vi "0 - Controle Xbox.vi"() -> (2 "R Thumb":i32(slide) scale=-32768.0..32768.0)   [LabVIEW 2020]
uses:
  <vilib>/robotics/Controls/Compass Indicator/Compass Indicator.xctl
  d73543a5-2c4f-4594-8cde-04c26e843dca.vi
  073897dc-bfc7-4ae1-a47e-8832abdac106.vi
  1fd616fa-7c11-4f18-9353-dc0f775eeb70.vi
  12afcf76-136b-4d38-a805-5952addfd333.vi
  20e97823-944d-452c-9f5c-32b38a6acdda.vi
  48340986-43e5-49c4-9512-bc3a2c788b05.vi
  cd7113f7-14d5-4977-ab3b-8115f77a9605.vi
  7e22e7d3-76e1-429a-a868-e97800e19938.vi
  749baf19-c05a-4ab2-9a75-a53bd8d5225c.vi
  9b3ce3fb-1892-4e24-a592-ce18c55ace7c.vi
  <vilib>/picture/3D Picture Control/Object/Create Object (drawable).vi
  <vilib>/Utility/inputDevices.llb/joystickAcquire.vi
  <vilib>/Utility/inputDevices.llb/closeJoystick.vi
  <vilib>/picture/3D Picture Control/NI_3D Picture Control.lvlib
panel:
  in  "Relative?":bool
  in  "Color":T1={"Red"=1.0, "Green"=0.0, "Blue"=0.0, "Alpha"=1.0}
  out "3D Picture":refnum<vi>(3d-picture)
  out "Garra Acionada":bool
  out "Slide 2":u8(slide) caption="Avanço da Garra" scale=0.0..100.0
  out "Slide":u8(slide) caption="Rotação"
  out "Altura 1":bool
  out "Altura 2":bool
  out "Altura 3":bool
  out "número 4":i32 caption="Y (apertar)"
  out "número 3":i32 caption="X (segurar)"
  out "número 2":i32 caption="B (soltar)"
  out "número":i32 caption="A (1-2-3)"
  out "Analógico Direito":dbl(xcontrol)
  out "Analógico Esquerdo":dbl(xcontrol)
  out "Start":bool
  out "Stop/Back":bool
  out "Right trigger":bool
  out "Left Trigger":bool
  out "Cluster":T2
  out "LThumb":i32(slide) scale=-32768.0..32768.0
  out "Left Thumb button":bool
  out "Right Thumb button":bool
  out "LB":bool
  out "RB":bool
  out "Y":bool
  out "X":bool
  out "B":bool
  out "A":bool caption="Boolean"
  out "joystick info":T3(array[cluster])
  out "direction info":T4
  out "button info":T5
  out "axis info":T6
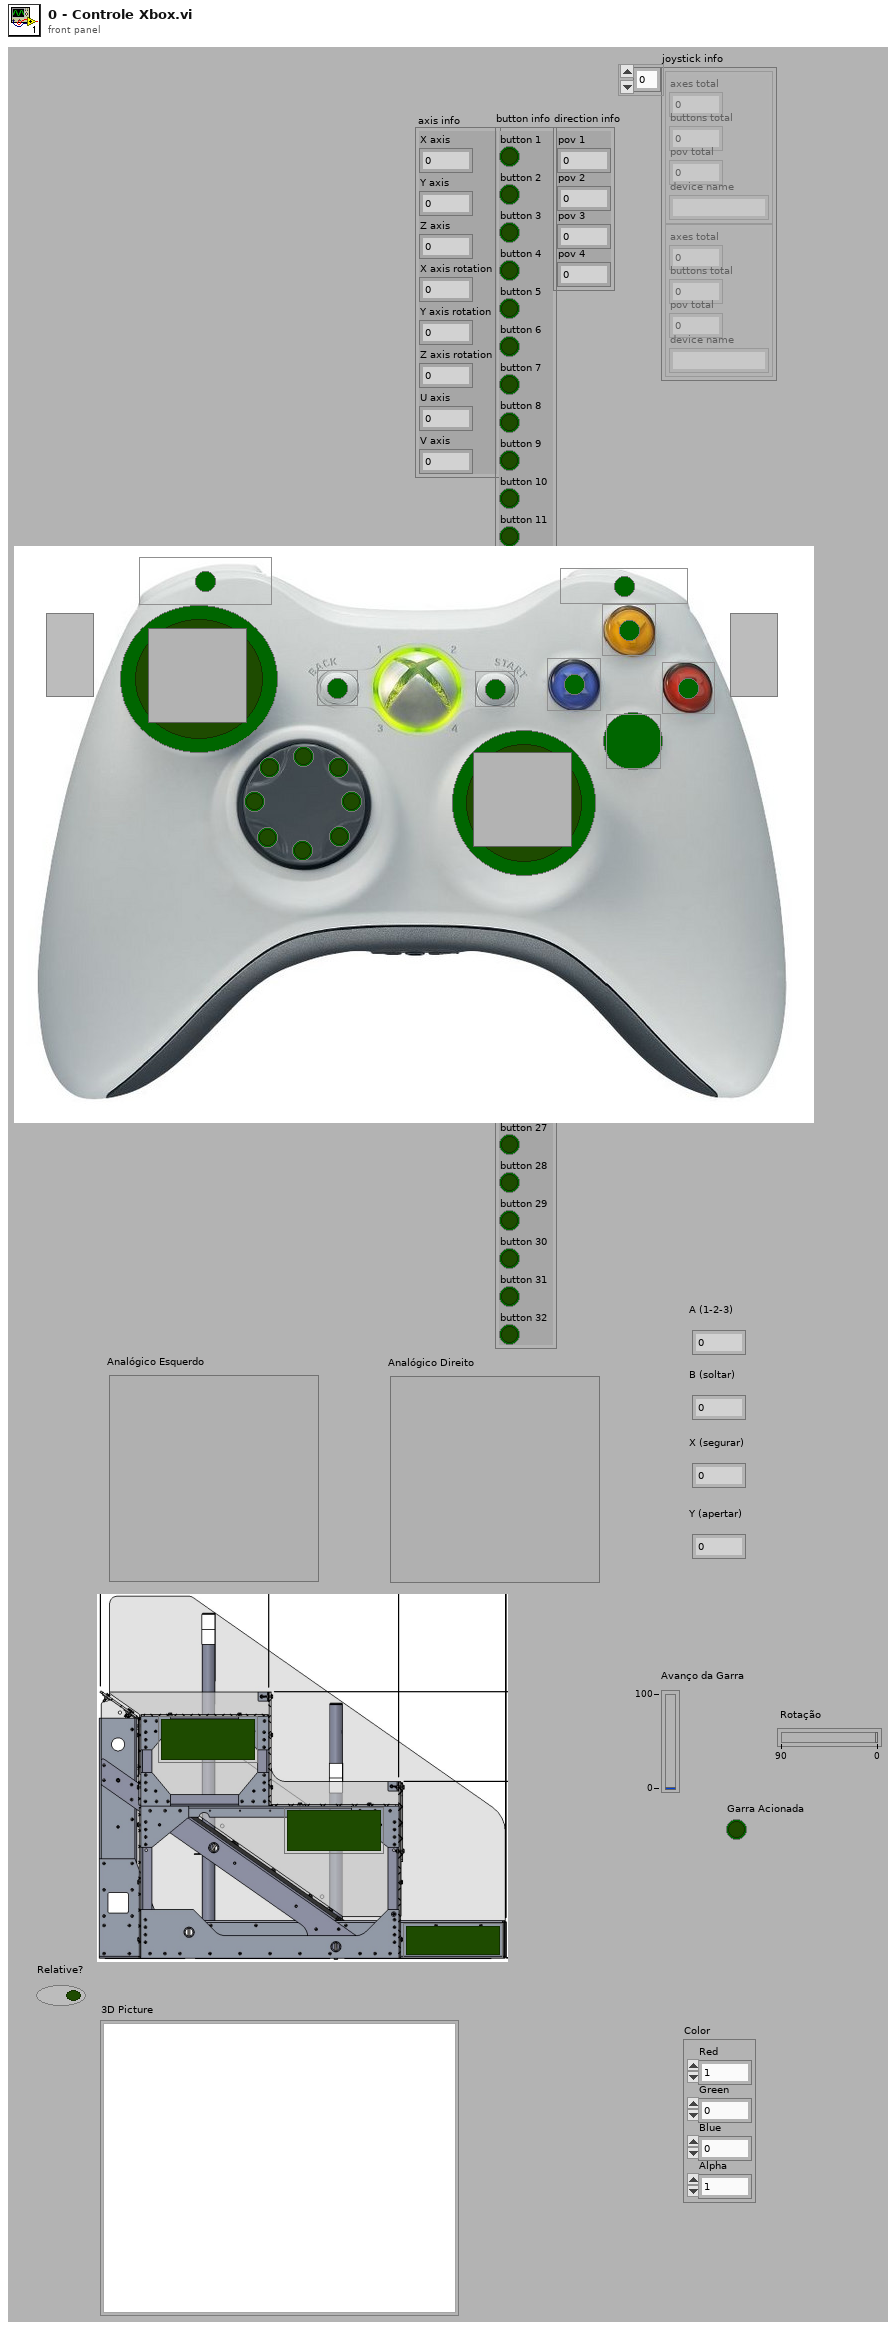
[diagram p1: front panel]
types:
  T1 = cluster{"Red":sgl, "Green":sgl, "Blue":sgl, "Alpha":sgl}
  T2 = cluster{"Boolean 4":bool, "Boolean 6":bool, "Boolean 3":bool, "Boolean 7":bool, "Boolean 2":bool, "Boolean 9":bool, "Boolean 5":bool, "Boolean 8":bool}
  T3 = cluster{"axes total":u32, "buttons total":u32, "pov total":u32, "device name":string}[]
  T4 = cluster{"pov 1":i32, "pov 2":i32, "pov 3":i32, "pov 4":i32}
  T5 = cluster{"button 1":bool, "button 2":bool, "button 3":bool, "button 4":bool, "button 5":bool, "button 6":bool, "button 7":bool, "button 8":bool, "button 9":bool, "button 10":bool, "button 11":bool, "button 12":bool, "button 13":bool, "button 14":bool, "button 15":bool, "button 16":bool, "button 17":bool, "button 18":bool, "button 19":bool, "button 20":bool, "button 21":bool, "button 22":bool, "button 23":bool, "button 24":bool, "button 25":bool, "button 26":bool, "button 27":bool, "button 28":bool, "button 29":bool, "button 30":bool, "button 31":bool, "button 32":bool}
  T6 = cluster{"X axis":i32, "Y axis":i32, "Z axis":i32, "X axis rotation":i32, "Y axis rotation":i32, "Z axis rotation":i32, "U axis":i32, "V axis":i32}
  T7 = cluster{"Array[0]":bool, "Array[1]":bool, "Array[2]":bool, "Array[3]":bool, "Array[4]":bool, "Array[5]":bool, "Array[6]":bool, "Array[7]":bool}
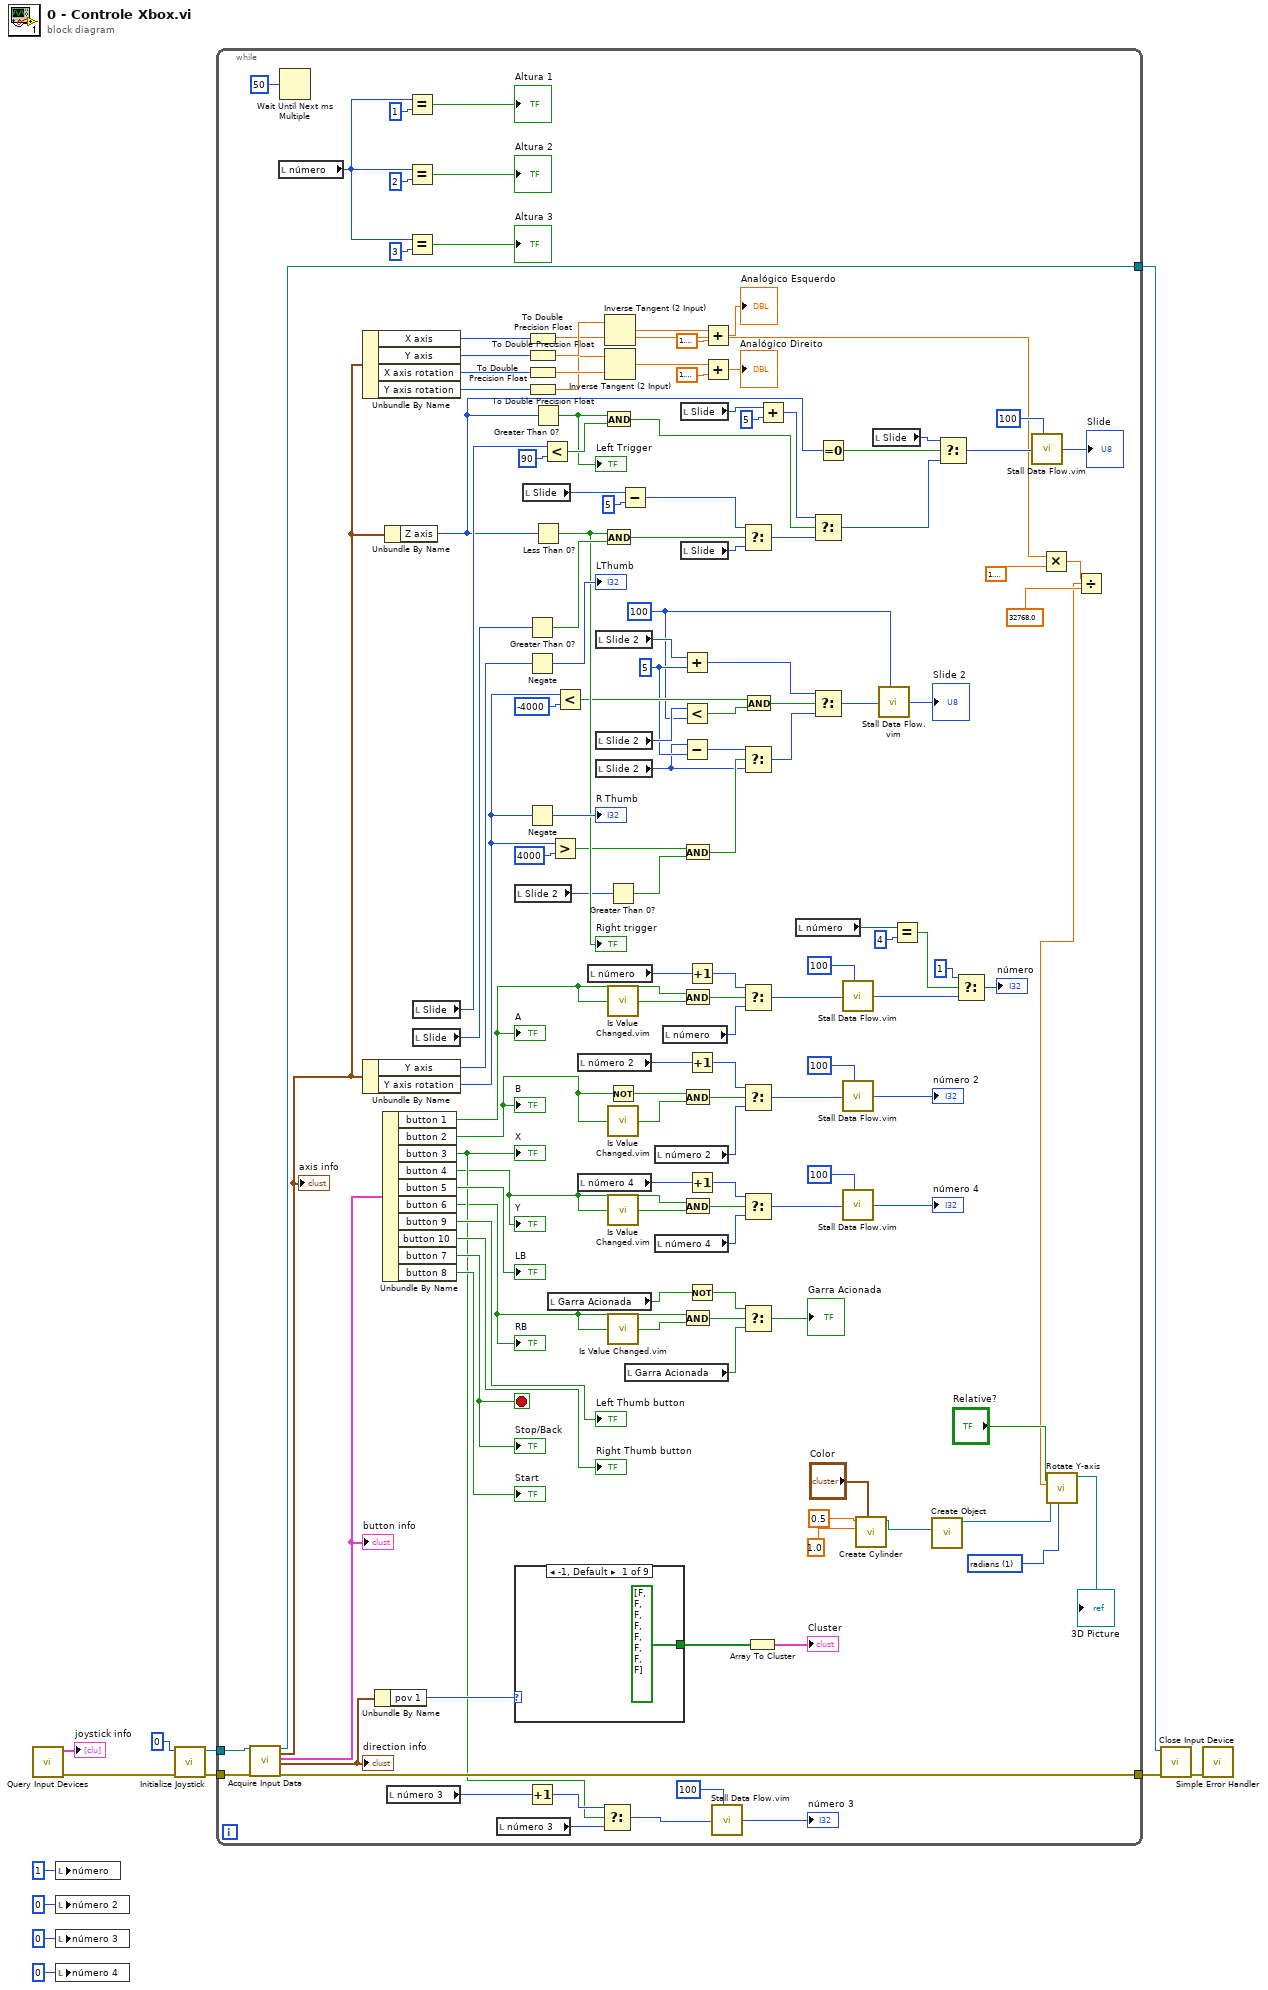
[diagram p0: block diagram]
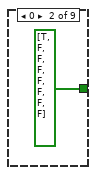
[diagram p2: hidden frame]
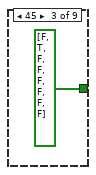
[diagram p3: hidden frame]
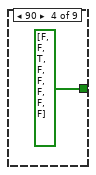
[diagram p4: hidden frame]
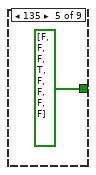
[diagram p5: hidden frame]
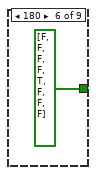
[diagram p6: hidden frame]
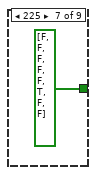
[diagram p7: hidden frame]
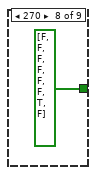
[diagram p8: hidden frame]
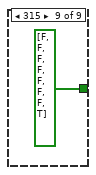
[diagram p9: hidden frame]
diagram:
  n1 = call <vilib>:"Query Input Devices.vi"() -> ("error out"=w6:errorcluster, "joystick info"=→"joystick info":T3)  [unwired: 1 in, 9 out]
  n2 = local write "número"(1) -> ()
  n3 = local write "número 2"(0) -> ()
  n4 = local write "número 3"(0) -> ()
  n5 = local write "número 4"(0) -> ()
  n6 = call <vilib>:"Initialize Joystick.vi"("error in (no error)"=w6, "device index"=0) -> ("error out"=w10:errorcluster, "device ID"=w11:refnum<k1>)  [unwired: 8 out]
  n7 = while {
    tunnel: w11 -> [w155]
    tunnel: w10 -> [w154]
    tunnel: [w153] -> w9
    tunnel: [w144] -> w8
    stop <- w142 stop-if-true
    w19 = u16 1 items=["degree", "radians"] ("angle unit")
    w38 = 5
    w34 = 100
    n8 = call-poly <vilib>:"Acquire Input Data.vi"("device ID"=w155, "error in (no error)"=w154) -> ("device ID"=w153:refnum<k1>, "axis info"=w134:T6, "button info"=w152:T5, "direction info"=w150:T4, "error out"=w144:errorcluster)  [unwired: 13 out]
    "axis info" <- w134
    "button info" <- w152
    "direction info" <- w150
    n9 = local read "número"() -> (w83:i32)
    n10 = Wait Until Next ms Multiple(millisecond multiple=u32 50) -> ()  [unwired: 1 out]
    n11 = Unbundle By Name(w134) -> ("X axis"=w136:i32, "Y axis"=w137:i32, "X axis rotation"=w67:i32, "Y axis rotation"=w79:i32)
    n12 = Unbundle By Name(w134) -> ("Y axis"=w139:i32, "Y axis rotation"=w44:i32)
    n13 = Unbundle By Name(w150) -> ("pov 1"=w149:i32)
    n14 = Unbundle By Name(w152) -> ("button 1"=w120:bool, "button 2"=w87:bool, "button 3"=w97:bool, "button 4"=w88:bool, "button 5"=→"LB":bool, "button 6"=w32:bool, "button 9"=→"Left Thumb button":bool, "button 10"=→"Right Thumb button":bool, "button 7"=w142:bool, "button 8"=→"Start":bool)
    "A" <- w120
    "B" <- w87
    "Y" <- w88
    "X" <- w97
    "RB" <- w32
    "Stop/Back" <- w142
    n15 = Unbundle By Name(w134) -> ("Z axis"=w60:i32)
    n16 = local read "número 3"() -> (w99:i32)
    n17 = Equal?(x=w83, y=1) -> (x = y?=→"Altura 1":bool)
    n18 = Equal?(x=w83, y=2) -> (x = y?=→"Altura 2":bool)
    n19 = Equal?(x=w83, y=3) -> (x = y?=→"Altura 3":bool)
    n20 = local read "Slide"() -> (w65:u8)
    n21 = local read "Slide"() -> (w78:u8)
    n22 = local read "número 3"() -> (w103:i32)
    n23 = local read "Slide 2"() -> (w42:u8)
    n24 = case shown="-1, Default" w149 {
      tunnel: [bool[] [FALSE, FALSE, FALSE, FALSE, FALSE, FALSE, FALSE, FALSE] ("Array") bool[] [TRUE, FALSE, FALSE, FALSE, FALSE, FALSE, FALSE, FALSE] ("Array") bool[] [FALSE, TRUE, FALSE, FALSE, FALSE, FALSE, FALSE, FALSE] ("Array") bool[] [FALSE, FALSE, TRUE, FALSE, FALSE, FALSE, FALSE, FALSE] ("Array") bool[] [FALSE, FALSE, FALSE, TRUE, FALSE, FALSE, FALSE, FALSE] ("Array") bool[] [FALSE, FALSE, FALSE, FALSE, TRUE, FALSE, FALSE, FALSE] ("Array") bool[] [FALSE, FALSE, FALSE, FALSE, FALSE, TRUE, FALSE, FALSE] ("Array") bool[] [FALSE, FALSE, FALSE, FALSE, FALSE, FALSE, TRUE, FALSE] ("Array") bool[] [FALSE, FALSE, FALSE, FALSE, FALSE, FALSE, FALSE, TRUE] ("Array")] -> w148
      frame -1, Default {
      }
      frame 0 {
      }
      frame 45 {
      }
      frame 90 {
      }
      frame 135 {
      }
      frame 180 {
      }
      frame 225 {
      }
      frame 270 {
      }
      frame 315 {
      }
    }
    n25 = local read "Slide"() -> (w74:u8)
    n26 = Greater Than 0?(x=w78) -> (x > 0?=w77:bool)
    n27 = Negate(x=w139) -> (-x=→"LThumb":i32)
    n28 = Negate(x=w44) -> (-x=→"R Thumb":i32)
    n29 = Increment(x=w99) -> (x+1=w98:i32)
    n30 = To Double Precision Float(number=w136) -> (double precision float=w17:dbl)
    n31 = To Double Precision Float(number=w137) -> (double precision float=w135:dbl)
    n32 = To Double Precision Float(number=w67) -> (double precision float=w131:dbl)
    n33 = To Double Precision Float(number=w79) -> (double precision float=w130:dbl)
    n34 = Greater Than 0?(x=w60) -> (x > 0?=w63:bool)
    "Left Trigger" <- w63
    n35 = Less Than 0?(x=w60) -> (x < 0?=w62:bool)
    "Right trigger" <- w62
    n36 = Less?(x=w65, y=90) -> (x < y?=w66:bool)
    n37 = local read "Garra Acionada"() -> (w29:bool)
    n38 = Greater?(x=w44, y=4000) -> (0:w40:bool)
    n39 = Less?(x=w44, y=-4000) -> (x < y?=w46:bool)
    n40 = local read "número 2"() -> (w113:i32)
    n41 = local read "número 4"() -> (w94:i32)
    n42 = local read "número"() -> (w124:i32)
    n43 = local read "Slide 2"() -> (w48:u8)
    n44 = local read "Slide 2"() -> (w50:u8)
    n45 = local read "Slide 2"() -> (w35:u8)
    n46 = Select(t=w98, s=w97, f=w103) -> (s? t:f=w102:i32)
    n47 = And(x=w63, y=w66) -> (x .and. y?=w71:bool)
    n48 = And(x=w62, y=w77) -> (x .and. y?=w76:bool)
    n49 = Inverse Tangent (2 Input)(1:w17, 2:w135) -> (0:w133:dbl)
    n50 = Inverse Tangent (2 Input)(1:w131, 2:w130) -> (0:w129:dbl)
    n51 = Greater Than 0?(x=w42) -> (x > 0?=w41:bool)
    n52 = call "Is Value Changed.vim"("value"=w120) -> ("changed or first call?"=w122:bool)
    n53 = Not(x=w87) -> (.not. x?=w111:bool)
    n54 = call "Is Value Changed.vim"("value"=w87) -> ("changed or first call?"=w115:bool)
    n55 = call "Is Value Changed.vim"("value"=w88) -> ("changed or first call?"=w92:bool)
    n56 = call "Is Value Changed.vim"("value"=w32) -> ("changed or first call?"=w33:bool)
    n57 = Subtract(x=w74, y=5) -> (x-y=w72:i32)
    n58 = local read "Garra Acionada"() -> (w27:bool)
    n59 = local read "número 2"() -> (w119:i32)
    n60 = local read "número 4"() -> (w95:i32)
    n61 = local read "número"() -> (w125:i32)
    n62 = local read "Slide"() -> (w69:u8)
    n63 = local read "Slide"() -> (w75:u8)
    n64 = Add(x=w48, y=w38) -> (x+y=w49:i32)
    n65 = Less?(x=w50, y=w34) -> (x < y?=w47:bool)
    n66 = Subtract(x=w35, y=w38) -> (x-y=w37:i32)
    n67 = And(x=w40, y=w41) -> (x .and. y?=w39:bool)
    n68 = And(x=w120, y=w122) -> (x .and. y?=w121:bool)
    n69 = And(x=w111, y=w115) -> (x .and. y?=w114:bool)
    n70 = And(x=w88, y=w92) -> (x .and. y?=w91:bool)
    n71 = And(x=w32, y=w33) -> (x .and. y?=w31:bool)
    n72 = Increment(x=w124) -> (x+1=w126:i32)
    n73 = Increment(x=w113) -> (x+1=w112:i32)
    n74 = Increment(x=w94) -> (x+1=w96:i32)
    n75 = Not(x=w29) -> (.not. x?=w28:bool)
    n76 = Add(x=w133, y=1.5707963267948966) -> (x+y=→"Analógico Esquerdo":dbl)
    n77 = Add(x=w129, y=1.5707963267948966) -> (x+y=→"Analógico Direito":dbl)
    n78 = call "Stall Data Flow.vim"("value in"=w102, "milliseconds to wait"=100) -> ("value out"=→"número 3":i32)  [unwired: 1 out]
    n79 = Select(t=w72, s=w76, f=w75) -> (s? t:f=w56:i32)
    n80 = Select(t=w37, s=w39, f=w35) -> (s? t:f=w36:i32)
    n81 = Select(t=w126, s=w121, f=w125) -> (s? t:f=w106:i32)
    n82 = Select(t=w112, s=w114, f=w119) -> (s? t:f=w118:i32)
    n83 = Select(t=w96, s=w91, f=w95) -> (s? t:f=w90:i32)
    n84 = Select(t=w28, s=w31, f=w27) -> (s? t:f=→"Garra Acionada":bool)
    n85 = And(x=w46, y=w47) -> (x .and. y?=w45:bool)
    n86 = Array To Cluster(array=w148) -> (cluster=→"Cluster":T7)
    n87 = Add(x=w69, y=5) -> (x+y=w68:i32)
    n88 = local read "número"() -> (w110:i32)
    n89 = Select(t=w68, s=w71, f=w56) -> (s? t:f=w54:i32)
    n90 = Select(t=w49, s=w45, f=w36) -> (s? t:f=w53:i32)
    n91 = Equal To 0?(x=w60) -> (x = 0?=w61:bool)
    n92 = call "Stall Data Flow.vim"("value in"=w106, "milliseconds to wait"=100) -> ("value out"=w105:i32)  [unwired: 1 out]
    n93 = call "Stall Data Flow.vim"("value in"=w118, "milliseconds to wait"=100) -> ("value out"=→"número 2":i32)  [unwired: 1 out]
    n94 = call "Stall Data Flow.vim"("value in"=w90, "milliseconds to wait"=100) -> ("value out"=→"número 4":i32)  [unwired: 1 out]
    n95 = call <vilib>:"Create Cylinder.vi"("Color"="Color", "Radius"=1.0, "Height"=0.5) -> ("New Cylinder Refnum"=w23:refnum<vi>)  [unwired: 7 in, 1 out]
    n96 = local read "Slide"() -> (w57:u8)
    n97 = call "Stall Data Flow.vim"("value in"=w53, "milliseconds to wait"=w34) -> ("value out"=→"Slide 2":i32)  [unwired: 1 out]
    n98 = Equal?(x=w110, y=4) -> (x = y?=w108:bool)
    n99 = call-poly <vilib>:"Create Object.vi"("Geometry"=w23) -> ("Scene:New Object"=w21:refnum<vi>)  [unwired: 9 in, 1 out]
    n100 = Select(t=w57, s=w61, f=w54) -> (s? t:f=w58:i32)
    n101 = Select(t=1, s=w108, f=w105) -> (s? t:f=→"número":i32)
    n102 = call "Stall Data Flow.vim"("value in"=w58, "milliseconds to wait"=100) -> ("value out"=→"Slide":i32)  [unwired: 1 out]
    n103 = Multiply(x=w17, y=1.5707963267948966) -> (x*y=w15:dbl)
    n104 = Divide(x=w15, y=32768.0) -> (x/y=w13:dbl)
    n105 = call <vilib>:"Rotate Y-axis.vi"("angle unit"=w19, "Relative?"="Relative?", "angle"=w13, "Scene Object In"=w21) -> ("Scene Object Out"=→"3D Picture":refnum<vi>)  [unwired: 6 in, 1 out]
  }
  n106 = call-poly <vilib>:"Close Input Device.vi"("error in (no error)"=w8, "device ID"=w9) -> ("error out"=w5:errorcluster)  [unwired: 8 out]
  n107 = call <vilib>:"Simple Error Handler.vi"("error in (no error)"=w5) -> ()  [unwired: 1 in, 8 out]
